vi "Build_Asylum_ShowVideo.vi"(8 "error in (no error)":errorcluster, 11 "Source":i32) -> (0 "error out":errorcluster, 3 "Command":string)   [LabVIEW 2020]
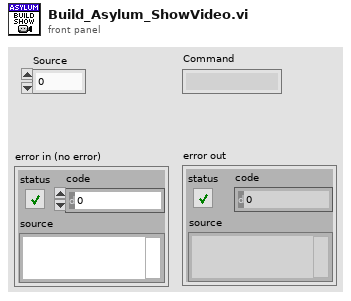
[diagram p1: front panel]
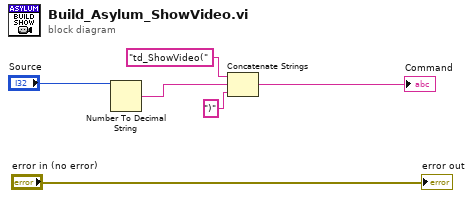
[diagram p0: block diagram]
diagram:
  n1 = Number To Decimal String(number="Source") -> (decimal integer string=w3:string)  [unwired: 1 in]
  n2 = Concatenate Strings("td_ShowVideo(" ("string"), w3, ")" ("string")) -> (→"Command":string)
  "error out" <- "error in (no error)"
